vi "McPherson Write & Read.vi"(4 "milliseconds to wait":u32, 5 "error in (no error)":errorcluster, 6 "Timeout Limit":dbl=0.5 format="%.2f", 7 "Write String":string="X\r", 8 "PortNumber":i32=1 min=0 max=5) -> (0 "error out":errorcluster, 1 "Timeout":bool, 2 "Error Out":bool, 3 "Read String\nshows:":string="XK= 3 I= 25078 V= 49152 \r\r\n")   [LabVIEW 2019]
doc: "Send commands to the McPherson 789A-3 controller and receive returned infomation.\n\nMcPherson 789A-3 controller Needs \"\\s\\r\" to initially respond! Then terminate commands with \"\\r\"\n\nThe Serial port number is a global variable."
uses:
  Serial Instruments/Serial Support VISA.llb/Serial Actions.ctl
  Globals and TypeDefs/Global Varibal Control.vi
panel:
  out "Read String":string="XK= 3 I= 25078 V= 49152 \r\r\n"
  # "Controller Needs \"\\s\\r\" to initially respond!  Then terminate commands with \"\\r\""
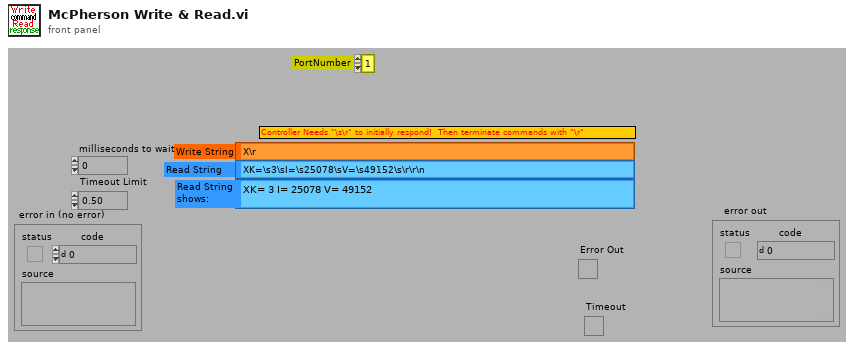
[diagram p1: front panel]
types:
  T1 = typedef "Serial Actions.ctl" = enum16{"Init", "Break", "Clear Buffer", "Write", "Read", "N Bytes", "Lock", "Unlock", "Close"}
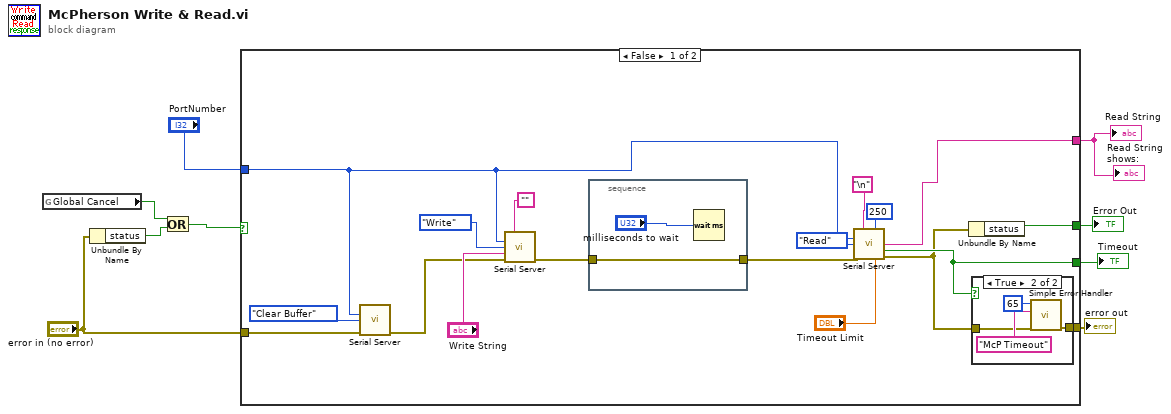
[diagram p0: block diagram]
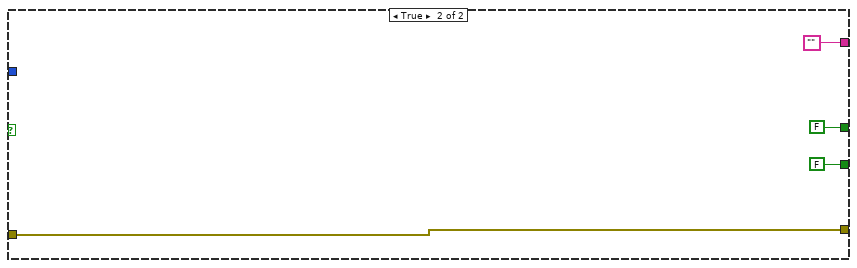
[diagram p3: hidden frame]
diagram:
  n1 = global read "Global Varibal Control.vi" "Global Cancel"() -> (w2:bool)
  n2 = Unbundle By Name("error in (no error)") -> ("status"=w3:bool)
  n3 = Or(x=w2, y=w3) -> (x .or. y?=w1:bool)
  n4 = case shown="False" w1 {
    tunnel: "error in (no error)" -> [w12 w38]
    tunnel: [w27 w38] -> w9
    tunnel: [w24 ""] -> w7
    tunnel: [w16 FALSE ("Error Out")] -> w6
    tunnel: [w18 FALSE ("Timeout")] -> w5
    tunnel: "PortNumber" -> [w11 _]
    frame False {
      n5 = call "Serial Server.vi"("Port Number"=w11, "Action"=Serial_Actions."Clear Buffer", "error in (no error)"=w12) -> ("error out"=w13:errorcluster)  [unwired: 8 in, 4 out]
      n6 = call "Serial Server.vi"("EOT Chars (cr/lf)"="", "Port Number"=w11, "Action"=Serial_Actions."Write", "String To Send"="Write String", "error in (no error)"=w13) -> ("error out"=w15:errorcluster)  [unwired: 6 in, 4 out]
      n7 = stacked-sequence {
        tunnel: [w29] -> w14
        tunnel: w15 -> [w29]
        frame #0 {
          n8 = Wait (ms)(milliseconds to wait="milliseconds to wait") -> ()  [unwired: 1 out]
        }
      }
      n9 = call "Serial Server.vi"("EOT Chars (cr/lf)"="\n", "Max Char to Read"=250, "Port Number"=w11, "Action"=Serial_Actions."Read", "error in (no error)"=w14, "Timeout Limit(sec)"="Timeout Limit") -> ("Serial Read"=w24:string, "Timeout"=w18:bool, "error out"=w17:errorcluster)  [unwired: 5 in, 2 out]
      n10 = Unbundle By Name(w17) -> ("status"=w16:bool)
      n11 = case shown="True" w18 {
        tunnel: w17 -> [w30 w32]
        tunnel: [w30 w31] -> w27
        frame False {
        }
        frame True {
          n12 = call <vilib>:"Simple Error Handler.vi"("error code (no error:0)"=65, "error source (\" \")"="McP Timeout", "error in (no error)"=w32) -> ("error out"=w31:errorcluster)  [unwired: 2 in, 4 out]
        }
      }
    }
    frame True {
    }
  }
  "error out" <- w9
  "Read String\nshows:" <- w7
  "Read String" <- w7
  "Timeout" <- w5
  "Error Out" <- w6
